vi "Pre Launch Init.vi"(11 "Calculadora in":refnum<class "Calculadora.lvclass">) -> (0 "error out":errorcluster, 3 "Calculadora out":refnum<class "Calculadora.lvclass">)   [LabVIEW 2020, in "Calculadora.lvlib" / "Calculadora.lvclass"]
doc: "(<B>Filename</B>: Actor Framework.lvlib:Actor.lvclass:Pre Launch Init.vi)\n\nDefines behavior that occurs after the Launch Nested Actor method is invoked but before the actor's Actor Core method begins running.\n\nBy default, this method does nothing. A descendant class may override it to define behavior."
uses:
  Calculadora.lvclass
  Calculadora.lvclass/Calculadora.ctl
  <vilib>/ActorFramework/Actor/Actor.lvclass
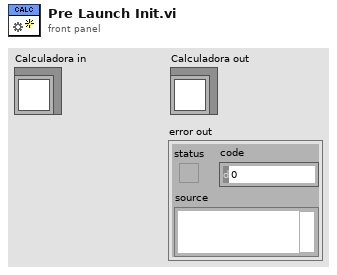
[diagram p1: front panel]
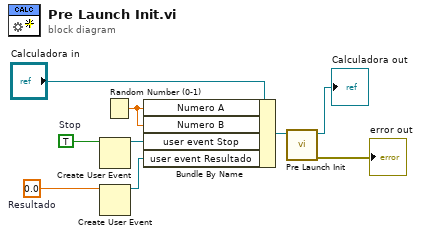
[diagram p0: block diagram]
diagram:
  w2 = 0.0  # Resultado
  w4 = TRUE  # Stop
  n1 = Create User Event(user event datatype=w4) -> (user event=w3:refnum<user-event>)  [unwired: 1 in, 1 out]
  n2 = Create User Event(user event datatype=w2) -> (user event=w1:refnum<user-event>)  [unwired: 1 in, 1 out]
  n3 = Random Number (0-1)() -> (number: 0 to 1=w5:dbl)
  n4 = Bundle By Name(cluster="Calculadora in", "Numero A"=w5, "Numero B"=w5, "user event Stop"=w3, "user event Resultado"=w1) -> (w6:refnum<class "Calculadora.lvclass">)
  n5 = call-parent "Pre Launch Init.vi"("Actor in"=w6) -> ("error out"=→"error out":errorcluster, "Actor out"=→"Calculadora out":refnum<class "Calculadora.lvclass">)  [unwired: 9 in]
